vi "Move From Output to Export Dir.vi"(0 "NI Build Specification in":refnum<class "NI Build Specification_LV.lvclass">, 11 "error IO":errorcluster) -> (4 "NI Build Specification out":refnum<class "NI Build Specification_LV.lvclass">, 15 "error out":errorcluster)   [LabVIEW 2017, in "CL_G3_VIComponentBuilder.lvlib" / "NI Build Specification_LV.lvclass"]
doc: "Each build specification of a LabVIEW Project defines an output directory where the build items are located. Subsequent builds know the location of the previous build outputs. This build output is a hardcoded path in the project. In order to be flexible, by convention, all build outputs are lcoated at C:\\builds\\<Export name>. This function moves the final built output to the export directory. It also moves the <Anchor><Text>temporary LabVIEW Project</Text><AnchorName>Create Temp Build Spec File Name</AnchorName><PageName>Export Class Documentation</PageName><Space>TCS</Space></Anchor> with the updated build numbers to the export directory."
uses:
  NI Build Specification_LV.lvclass
  C:/builds/Component BuilderBT/SrcDist/Exports/Exports/Export.lvclass
  Exports/Export.lvclass/Export.ctl
  Exports/Accessors/Read Exported Build Specification Path.vi
  Exports/Accessors/Read Component Export Dir.vi
  Exports/Accessors/Read Export Build Specification.vi
  Exports/Accessors/Write Exported Build Specification Path.vi
  Exports/Accessors/Write Export Operation Errors.vi
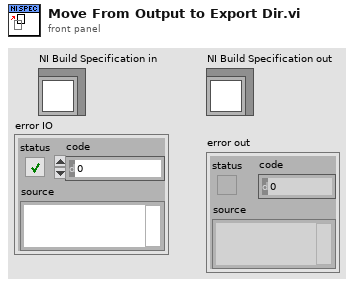
[diagram p1: front panel]
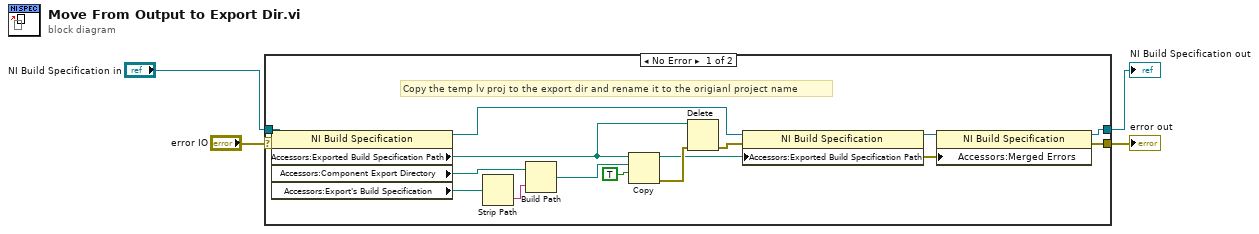
[diagram p0: block diagram]
diagram:
  n1 = case shown="No Error" "error IO" {
    selector: "error IO" -> [w8 w22]
    tunnel: [w7 w22] -> w3
    tunnel: "NI Build Specification in" -> [w11 w21]
    tunnel: [w9 w21] -> w2
    frame No Error {
      # "Copy the temp lv proj to the export dir and rename it to the origianl project name"
      n2 = property class="NI Build Specification"(reference=w11, error in=w8) -> (reference out=w19:refnum<class "NI Build Specification_LV.lvclass">, "Accessors:Exported Build Specification Path"=w5:path, "Accessors:Component Export Directory"=w13:path, "Accessors:Export's Build Specification"=w18:path)  [unwired: 1 out]
      n3 = Strip Path(path=w18) -> (name=w17:string)  [unwired: 1 out]
      n4 = Build Path(base path=w13, name or relative path=w17) -> (appended path=w16:path)
      n5 = Copy(9:TRUE ("overwrite (F)"), 10:w16, 11:w5) -> (0:w15:errorcluster, 3:w12:path)  [unwired: 2 in, 1 out]
      n6 = Delete(path (use dialog)=w5, error in=w15) -> (error out=w14:errorcluster)  [unwired: 3 in, 2 out]
      n7 = property class="NI Build Specification"(reference=w19, error in=w14, "Accessors:Exported Build Specification Path"=w12) -> (reference out=w10:refnum<class "NI Build Specification_LV.lvclass">, error out=w6:errorcluster)
      n8 = property class="NI Build Specification"(reference=w10, "Accessors:Merged Errors"=w6) -> (reference out=w9:refnum<class "NI Build Specification_LV.lvclass">, error out=w7:errorcluster)  [unwired: 1 in]
    }
    frame Error {
    }
  }
  "error out" <- w3
  "NI Build Specification out" <- w2
